vi "increment error.vi"(8 "error in (no error)":errorcluster, 11 "Master CR in":refnum<class "WebSocket Client CR.lvclass">) -> (0 "error out":errorcluster, 2 "N errors":i32, 3 "Master CR out":refnum<class "WebSocket Client CR.lvclass">)   [LabVIEW 2021, in "WebSockets.lvlib" / "WebSocket Client CR.lvclass"]
uses:
  WebSocket Client CR.lvclass
  WebSocket Client CR.lvclass/WebSocket Client CR.ctl
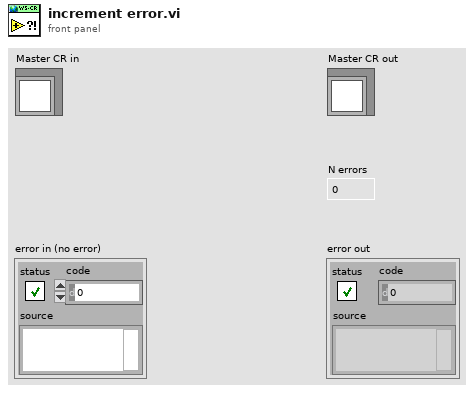
[diagram p1: front panel]
types:
  T1 = typedef "WebSockets.lvlib/WebSocket Client CR.lvclass/Master CR state.ctl" = cluster{"state":T2, "enable":bool, "write enable":bool, "connect":bool, "errors":i32, "Run":bool, "Write":bool, "Stop":bool}
  T2 = typedef "WebSockets.lvlib/WebSocket Client CR.lvclass/CR_Core_State.ctl" = enum8{"initialization", "redefine", "standby", "ping", "connect", "wait to reconnect", "wait to reset timeout", "configure", "requests", "close connection", "stop"}
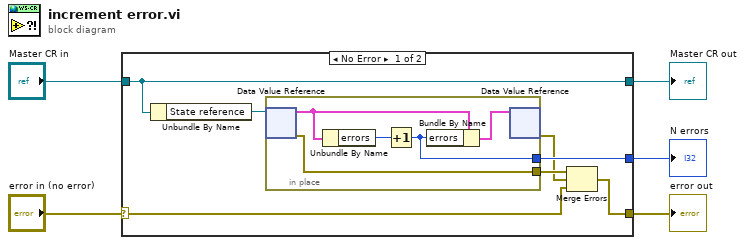
[diagram p0: block diagram]
diagram:
  n1 = case shown="No Error" "error in (no error)" {
    selector: "error in (no error)" -> [w7 w18]
    tunnel: [w6 w18] -> w1
    tunnel: [w10 w19] -> w4
    tunnel: "Master CR in" -> [w10 w19]
    tunnel: [w12 _] -> w2
    frame No Error {
      n2 = Unbundle By Name(w10) -> ("State reference"=w11:refnum<data-value>)
      n3 = in-place {
        in-place-border: [w14] -> w12
        in-place-border: [w13] -> w9
        n4 = in-place-dvr #1(w11) -> (w16:T1, w13:errorcluster)
        n5 = Unbundle By Name(w16) -> ("errors"=w17:i32)
        n6 = Increment(x=w17) -> (x+1=w14:i32)
        n7 = Bundle By Name(cluster=w16, "errors"=w14) -> (w15:T1)
        n8 = in-place-dvr #1(w15) -> (w8:errorcluster)  [unwired: 1 out]
      }
      n9 = Merge Errors(w9, w8, w7) -> (w6:errorcluster)
    }
    frame Error {
    }
  }
  "error out" <- w1
  "Master CR out" <- w4
  "N errors" <- w2
